vi "Orion PDU Rd Wr settings json.vi"(7 "Name":string, 8 "error in (no error)":errorcluster, 9 "Settings File":string="CC System Settings.json", 10 "Write? (F:Read)":bool, 11 "Orion Parameters":T1) -> (0 "error out":errorcluster, 3 "Orion Parameters":T1)   [LabVIEW 2024, in "Orion PDU.lvclass"]
uses:
  Orion PDU.lvclass
  typedef Orion PDU Settings.ctl
  2e80df6d-94aa-46b9-8b94-ceea8c057880.vi
  659fb017-0e9f-42f9-b06e-930303f00cbc.vi
  <vilib>/JDP Science/JSONtext/Find Item.vi
  <vilib>/JDP Science/JSONtext/Next JSON Value.vi
  <vilib>/JDP Science/JSONtext/String Subset.vi
  <vilib>/JDP Science/JSONtext/Parsing/Advance past next JSON Value (inlined COPY).vi
  <vilib>/JDP Science/JSONtext/Parsing/Advance past whitespace.vi
  <vilib>/JDP Science/JSONtext/Parsing/Advance past String.vi
  <vilib>/JDP Science/JSONtext/Parsing/Advance past Number.vi
  <vilib>/JDP Science/JSONtext/Parsing/Advance past Line Ending.vi
  <vilib>/JDP Science/JSONtext/Parsing/Parse Full Path or Item Name.vi
  <vilib>/JDP Science/JSONtext/Parsing/Advance past Array.vi
  <vilib>/JDP Science/JSONtext/Parsing/Advance past Object.vi
  <vilib>/JDP Science/JSONtext/support/Error Cluster From Code.vi
  <vilib>/JDP Science/JSONtext/Offset/Find Item Locations by Path.vi
  <vilib>/JDP Science/JSONtext/JSON text to Variant.vi
  <vilib>/JDP Science/JSONtext/Variant to JSON Text.vi
  <vilib>/JDP Science/JSONtext/Set Item.vi
  <vilib>/JDP Science/JSONtext/LVClass Serializer/JSONtext LVClass Serializer.lvclass
  Orion PDU.lvclass/Orion PDU.ctl
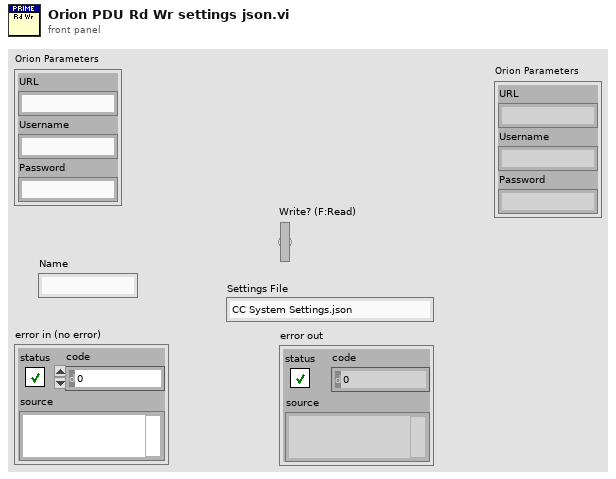
[diagram p1: front panel]
types:
  T1 = typedef "Orion PDU.lvclass/typedef Orion PDU Settings.ctl" = cluster{"URL":string, "Username":string, "Password":string}
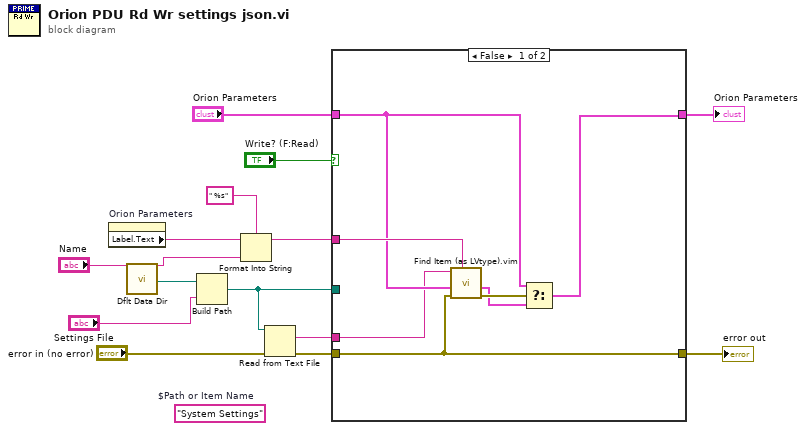
[diagram p0: block diagram]
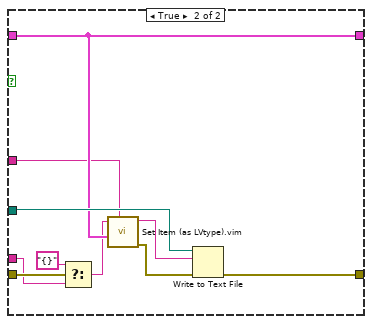
[diagram p2: hidden frame]
diagram:
  (unwired) "System Settings"  # $Path or Item Name
  n1 = property on="Orion Parameters" class="Clust (strict)"() -> ("Label.Text"=w4:string)  [unwired: 2 in, 2 out]
  n2 = call <vilib>:"Dflt Data Dir.vi"() -> ("App:Default Data Directory"=w11:path)
  n3 = Build Path(base path=w11, name or relative path="Settings File") -> (appended path=w5:path)
  n4 = Format Into String(format string=" %s", initial string=w4, "Name") -> (resulting string=w3:string)  [unwired: 1 in, 1 out]
  n5 = Read from Text File(file (use dialog)=w5, error in="error in (no error)") -> (text=w6:string, error out=w7:errorcluster)  [unwired: 2 in, 2 out]
  n6 = case shown="False" "Write? (F:Read)" {
    tunnel: w7 -> [w15 w26]
    tunnel: "Orion Parameters" -> [w19 w29]
    tunnel: w5 -> [_ w31]
    tunnel: [w15 w30] -> w10
    tunnel: [w21 w29] -> w9
    tunnel: w3 -> [w20 w28]
    tunnel: w6 -> [w16 w24]
    frame False {
      n7 = call "Find Item (as LVtype).vim"("$Path or Item Name"=w20, "error in (no error)"=w15, "Data Type and Default Value"=w19, "JSON"=w16) -> ("error out"=w18:errorcluster, "Data"=w17:T1)  [unwired: 4 in, 2 out]
      n8 = Select(t=w19, s=w18, f=w17) -> (s? t:f=w21:T1)
    }
    frame True {
      n9 = Select(t="{}" ("JSON"), s=w26, f=w24) -> (s? t:f=w23:string)
      n10 = call "Set Item (as LVtype).vim"("$Path or Item Name"=w28, "Anything"=w29, "JSON"=w23) -> ("error out"=w22:errorcluster, "<JSON>"=w27:string)  [unwired: 5 in, 1 out]
      n11 = Write to Text File(file (use dialog)=w31, text=w27, error in=w22) -> (error out=w30:errorcluster)  [unwired: 1 in, 2 out]
    }
  }
  "error out" <- w10
  "Orion Parameters" <- w9
